vi "Create Path.vi"(8 "error in (no error)":errorcluster) -> (0 "error out":errorcluster, 3 "File Path Control":path)   [LabVIEW 2016, in "Logger.lvlib"]
uses:
  Logger.lvlib
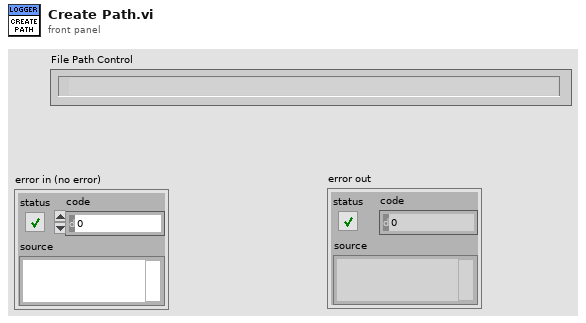
[diagram p1: front panel]
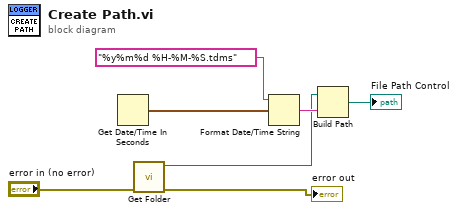
[diagram p0: block diagram]
diagram:
  n1 = Get Date/Time In Seconds() -> (seconds since 1Jan1904=w7:timestamp)
  n2 = call "Get Folder.vi"("error in (no error)"="error in (no error)") -> ("error out"=→"error out":errorcluster, "dup path"=w3:path)  [unwired: 9 in]
  n3 = Format Date/Time String(time format string (%c)="%y%m%d %H-%M-%S.tdms", seconds (now)=w7) -> (date/time string=w5:string)  [unwired: 1 in]
  n4 = Build Path(base path=w3, name or relative path=w5) -> (appended path=→"File Path Control":path)
